vi "ReadWriteParamPLC.vi"(8 "error in (no error)":errorcluster, 11 "StepMotor in":refnum<class "StepMotor.lvclass">) -> (0 "error out":errorcluster, 3 "StepMotor out":refnum<class "StepMotor.lvclass">)   [LabVIEW 2010, in "StepMotor.lvclass"]
doc: "Формирование сообщения для последующей записи в привод СПШ"
uses:
  StepMotor.lvclass
  StepMotor.lvclass/StepMotor.ctl
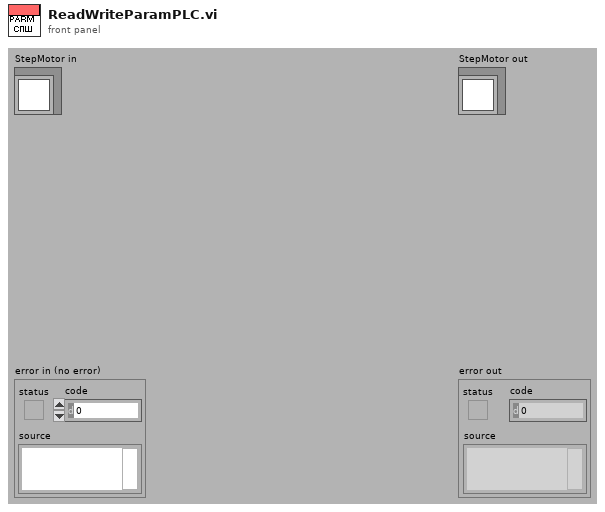
[diagram p1: front panel]
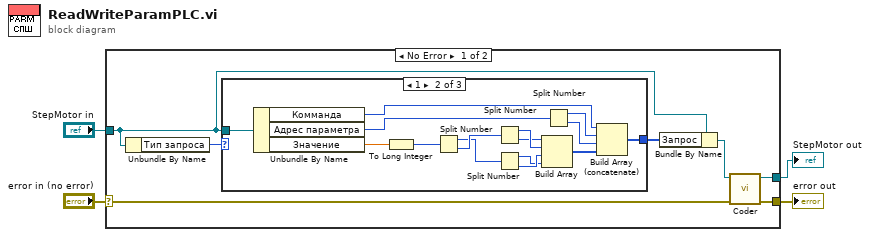
[diagram p0: block diagram]
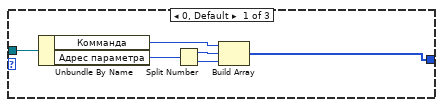
[diagram p2: hidden frame]
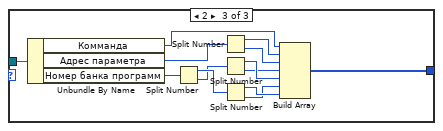
[diagram p3: hidden frame]
diagram:
  n1 = case shown="No Error" "error in (no error)" {
    selector: "error in (no error)" -> [w9 w47]
    tunnel: [w8 w47] -> w3
    tunnel: [w5 w46] -> w1
    tunnel: "StepMotor in" -> [w7 w46]
    frame No Error {
      n2 = Unbundle By Name(w7) -> ("Тип запроса"=w6:u16)
      n3 = case shown="1" w6 {
        tunnel: [w17 w32 w45] -> w11
        tunnel: w7 -> [w16 w30 w44]
        frame 0, Default {
          n4 = Unbundle By Name(w16) -> ("Комманда"=w14:u8, "Адрес параметра"=w15:u16)
          n5 = Split Number(x=w15) -> (hi(x)=w13:u8, lo(x)=w12:u8)
          n6 = Build Array(w14, w13, w12) -> (w17:u8[])
        }
        frame 1 {
          n7 = Unbundle By Name(w30) -> ("Комманда"=w20:u8, "Адрес параметра"=w29:u16, "Значение"=w19:dbl)
          n8 = To Long Integer(number=w19) -> (32bit integer=w18:i32)
          n9 = Split Number(x=w18) -> (hi(x)=w27:u16, lo(x)=w28:u16)
          n10 = Split Number(x=w28) -> (hi(x)=w24:u8, lo(x)=w23:u8)
          n11 = Split Number(x=w27) -> (hi(x)=w25:u8, lo(x)=w26:u8)
          n12 = Build Array(w23, w24, w26, w25) -> (w31:u8[])
          n13 = Split Number(x=w29) -> (hi(x)=w22:u8, lo(x)=w21:u8)
          n14 = Build Array (concatenate)(w20, w22, w21, w31) -> (w32:u8[])
        }
        frame 2 {
          n15 = Unbundle By Name(w44) -> ("Комманда"=w40:u8, "Адрес параметра"=w43:u16, "Номер банка программ"=w37:u16)
          n16 = Split Number(x=w37) -> (hi(x)=w39:u8, lo(x)=w38:u8)
          n17 = Split Number(x=w43) -> (hi(x)=w42:u8, lo(x)=w41:u8)
          n18 = Split Number(x=w38) -> (hi(x)=w34:u8, lo(x)=w33:u8)
          n19 = Split Number(x=w39) -> (hi(x)=w36:u8, lo(x)=w35:u8)
          n20 = Build Array(w40, w42, w41, w33, w34, w35, w36) -> (w45:u8[])
        }
      }
      n21 = Bundle By Name(cluster=w7, "Запрос"=w11) -> (w10:refnum<class "StepMotor.lvclass">)
      n22 = call "Coder.vi"("error in (no error)"=w9, "StepMotor in"=w10) -> ("error out"=w8:errorcluster, "StepMotor out"=w5:refnum<class "StepMotor.lvclass">)  [unwired: 8 in]
    }
    frame Error {
    }
  }
  "error out" <- w3
  "StepMotor out" <- w1
